vi "PH_Stepmotor_BaseClass.set Device Error.vi"(0 "i ref in":refnum<vi>, 4 "Device Error":errorcluster, 5 "error in":errorcluster) -> (14 "i ref out":refnum<vi>, 19 "error out":errorcluster)   [LabVIEW 2014, in "PH_Stepmotor_BaseClass.lvlib"]
doc: "This VI compares the incoming device error with the one stored one in own attributes; if different, the new value is stored."
uses:
  PH_Stepmotor_BaseClass.lvlib
  PH_Common/PH_Common.lvlib
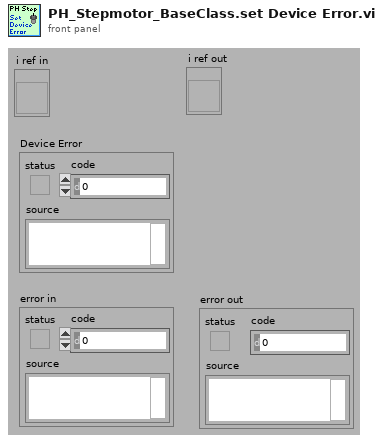
[diagram p1: front panel]
types:
  T1 = typedef "PH_Stepmotor_BaseClass.lvlib/PH_Stepmotor_BaseClass.i attribute.ctl" = cluster{"Device Error":errorcluster, "Axes PSDB Thread":cluster{"Ref":refnum<vi>, "Q-Ref":refnum<queue>, "Data Status":T2}, "Axes":T3[], "Axes PSDB Infos":cluster{"GUI Name":string, "PSDB Instance ID":i32, "PSDB Status Service ID":i32, "Axis":i32, "Class":string}[], "GUI Refs":T8}
  T2 = typedef "PH_PSDBWriter.lvlib/PH_PSDBWriter.Data Status.ctl" = i16
  T3 = typedef "PH_Stepmotor_BaseClass.lvlib/PH_Stepmotor_BaseClass.Axis Attributes.ctl" = cluster{"Settings":T4, "Endswitch?":bool, "DIM Service IDs":T6, "Activity":T7, "Configured?":bool, "Position":cluster{"Current":i32, "Target":i32}, "Position to set":cluster{"New?":bool, "Wanted":i32}, "Stop?":bool, "Reset?":bool, "Move?":bool, "Nothing connected?":bool}
  T4 = typedef "PH_Stepmotor_BaseClass.lvlib/PH_Stepmotor_BaseClass.Axis Settings.ctl" = cluster{"Sign change":bool, "Width":dbl, "Calibration":dbl, "Unit":string, "Motor Type":T5, "Unit Width":string, "Unit CF":string}
  T5 = typedef "PH_Stepmotor_BaseClass.lvlib/PH_Stepmotor_BaseClass.Motor Type.ctl" = enum16{"Unspecific", "OWIS 49.120.2633", "OWIS 49.060.1033", "OWIS 43.040.2558", "Diamond Motion 2200 series", "OWIS 49.120.266B.MV6", "Calorimeter", "Linear Stage 1", "MICOS VT-80", "MICOS VT-80 S", "Standa Rotstage nt0.95A", "PUF RA 320.200", "PUF RA 800.200", "PUF RA 800.400", "PUF RA 400.50", "1324.nn.800.50", "1324.n9c.800.50", "1324.nn.320.200", "1324.nn.400.200", "1324.nn.800.200", "1324.nn.400.50", "1324.8c9c.800.50", "1324.8c9c.400.200"}
  T6 = typedef "PH_Stepmotor_BaseClass.lvlib/PH_Stepmotor_BaseClass.Axis DIM Service IDs.ctl" = cluster{"Settings":i32, "Information":i32}
  T7 = typedef "PH_Stepmotor_BaseClass.lvlib/PH_Stepmotor_BaseClass.Axis Activity.ctl" = enum16{"No Information", "stopped", "running", "Failure", "Alarm", "stopped at backward ES", "stopped at foreward ES"}
  T8 = typedef "PH_Stepmotor_BaseClass.lvlib/PH_Stepmotor_BaseClass.GUI Refs.ctl" = cluster{"Axes Configuration":refnum<vi>, "Device Error":refnum<vi>, "Axes PSDB Infos":refnum<vi>}
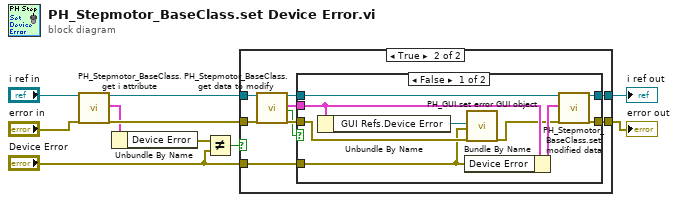
[diagram p0: block diagram]
diagram:
  n1 = call "PH_Stepmotor_BaseClass.get i attribute.vi"("i ref in"="i ref in", "error in (no error)"="error in") -> ("i ref out"=w9:refnum<vi>, "i attribute"=w4:T1, "error out"=w7:errorcluster)  [unwired: 15 in]
  n2 = Unbundle By Name(w4) -> ("Device Error"=w3:errorcluster)
  n3 = Not Equal?(x=w3, y="Device Error") -> (x != y?=w1:bool)
  n4 = case shown="True" w1 {
    tunnel: [w11 w20] -> w10
    tunnel: w9 -> [w12 w17]
    tunnel: [w12 w16] -> w8
    tunnel: w7 -> [w11 w15]
    tunnel: "Device Error" -> [_ w14]
    frame False {
    }
    frame True {
      n5 = call "PH_Stepmotor_BaseClass.get data to modify.vi"("i ref in"=w17, "error in (no error)"=w15) -> ("i ref out"=w18:refnum<vi>, "i attribute"=w21:T1, "timed out"=w13:bool, "error out"=w19:errorcluster)  [unwired: 14 in]
      n6 = case shown="False" w13 {
        tunnel: w21 -> [w26 _]
        tunnel: [w29 w31] -> w20
        tunnel: w19 -> [w25 w31]
        tunnel: w18 -> [w28 w32]
        tunnel: [w27 w32] -> w16
        tunnel: w14 -> [w22 _]
        frame False {
          n7 = Unbundle By Name(w26) -> ("GUI Refs.Device Error"=w23:refnum<vi>)
          n8 = Bundle By Name(cluster=w26, "Device Error"=w22) -> (w30:T1)
          n9 = call "PH_GUI.set error GUI object.vi"("GUI Refs.Device Error"=w23, "error to set"=w22, "error in (no error)"=w25) -> ("error out"=w24:errorcluster)  [unwired: 16 in]
          n10 = call "PH_Stepmotor_BaseClass.set modified data.vi"("i ref in"=w28, "i attribute"=w30, "error in (no error)"=w24) -> ("i ref out"=w27:refnum<vi>, "error out"=w29:errorcluster)  [unwired: 15 in]
        }
        frame True {
        }
      }
    }
  }
  "error out" <- w10
  "i ref out" <- w8
